vi "InitPiece.vi"(8 "error in (no error)":errorcluster, 11 "object in":refnum<class "King.lvclass">) -> (0 "error out":errorcluster, 3 "object out":refnum<class "King.lvclass">)   [LabVIEW 2020, in "King.lvclass"]
uses:
  King.lvclass
  C:/_repos/_personal/Chess/Chess_LV/source/Pieces/Piece.lvclass
  typedefs/pieceType.ctl
  King.lvclass/King.ctl
  Piece.lvclass
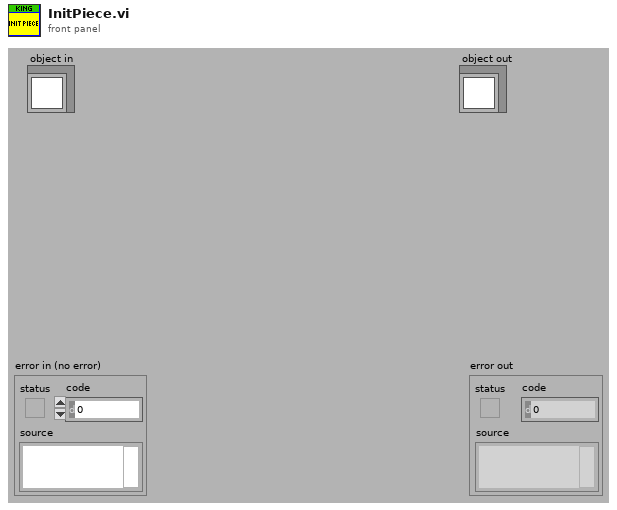
[diagram p1: front panel]
types:
  T1 = typedef "Piece.lvclass/pieceType.ctl" = enum16{"K", "Q", "R", "N", "B", "P", "none"}
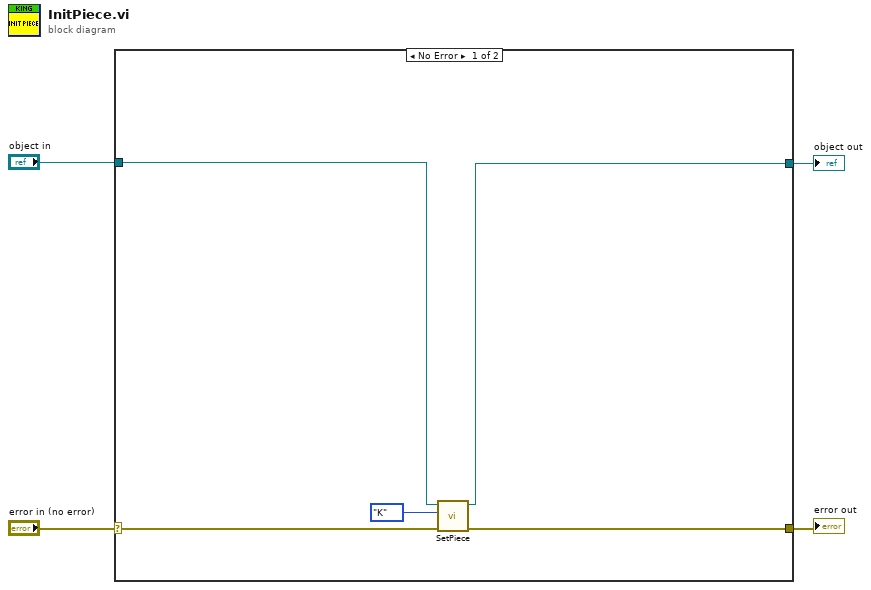
[diagram p0: block diagram]
diagram:
  n1 = case shown="No Error" "error in (no error)" {
    selector: "error in (no error)" -> [w9 w11]
    tunnel: [w8 w11] -> w3
    tunnel: [w6 w10] -> w1
    tunnel: "object in" -> [w7 w10]
    frame No Error {
      n2 = call "SetPiece.vi"("error in (no error)"=w9, "piece"=pieceType."K", "object in"=w7) -> ("error out"=w8:errorcluster, "object out"=w6:refnum<class "King.lvclass">)  [unwired: 7 in]
    }
    frame Error {
    }
  }
  "error out" <- w3
  "object out" <- w1
